vi "GetType.vi"(8 "error in (no error)":errorcluster, 11 "Configure AM Internal [AM] Msg":refnum<class "Configure AM Internal [AM] Msg.lvclass">) -> (0 "error out":errorcluster, 2 "Data Sample":variant, 3 "Configure AM Internal [AM] Msg":refnum<class "Configure AM Internal [AM] Msg.lvclass">)   [LabVIEW 2015, in "CS++Fgen.lvlib" / "Configure AM Internal [AM] Msg.lvclass"]
doc: "This VI delivers a sample of the data type format the message expects."
uses:
  Configure AM Internal [AM] Msg.lvclass
  Configure AM Internal [AM] Msg.lvclass/Configure AM Internal [AM] Msg.ctl
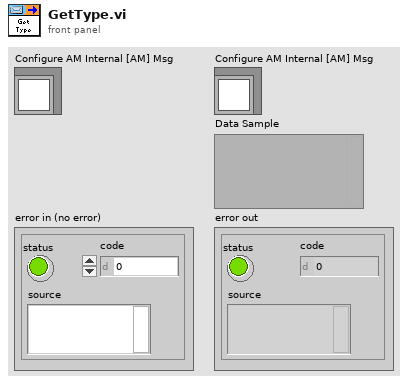
[diagram p1: front panel]
types:
  T1 = cluster{"modulation depth (0.00 %)":dbl, "modulation frequency (1000 Hz)":dbl[unit], "modulation waveform (Sine)":i32}
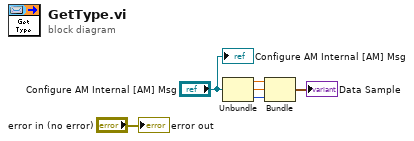
[diagram p0: block diagram]
diagram:
  n1 = Unbundle("Configure AM Internal [AM] Msg") -> (w3:dbl, w2:dbl[unit], w1:i32)
  n2 = Bundle("modulation depth (0.00 %)"=w3, "modulation frequency (1000 Hz)"=w2, "modulation waveform (Sine)"=w1) -> (→"Data Sample":T1)  [unwired: 1 in]
  "error out" <- "error in (no error)"
  "Configure AM Internal [AM] Msg" <- "Configure AM Internal [AM] Msg"
